vi "GSP_GUI_user.vi"(4 "error in":errorcluster, 7 "User File":path) -> (0 "error out":errorcluster, 1 "User Type":T1, 2 "Canceled?":bool)   [LabVIEW 2015]
doc: "A login GUI that reads and validates from the supplied user INI file"
uses:
  GUI_states.ctl
  GSP_GUI_global.vi
panel:
  out "Status":string
  in  "OK Button":bool
  in  "Password":string
  in  "Known Users":u16(ring) items=["barlow", "operators", "fraga", "rosteen", "clemens", "heathcote", "points", "unc", "msu", "brazil", "noao"]
  # "Welcome to the Goodman Spectrograph Control System. Please Select your username to the right or enter a a new name and press \"OK\""
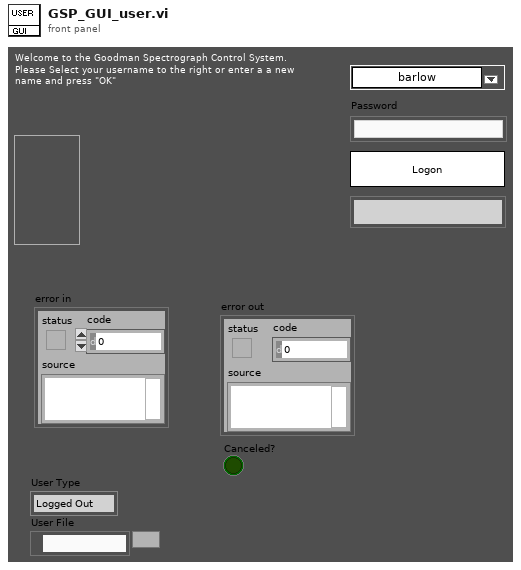
[diagram p1: front panel]
types:
  T1 = typedef "GUI_states.ctl" = enum16{"Logged Out", "Observer", "Operator", "Engineer"}
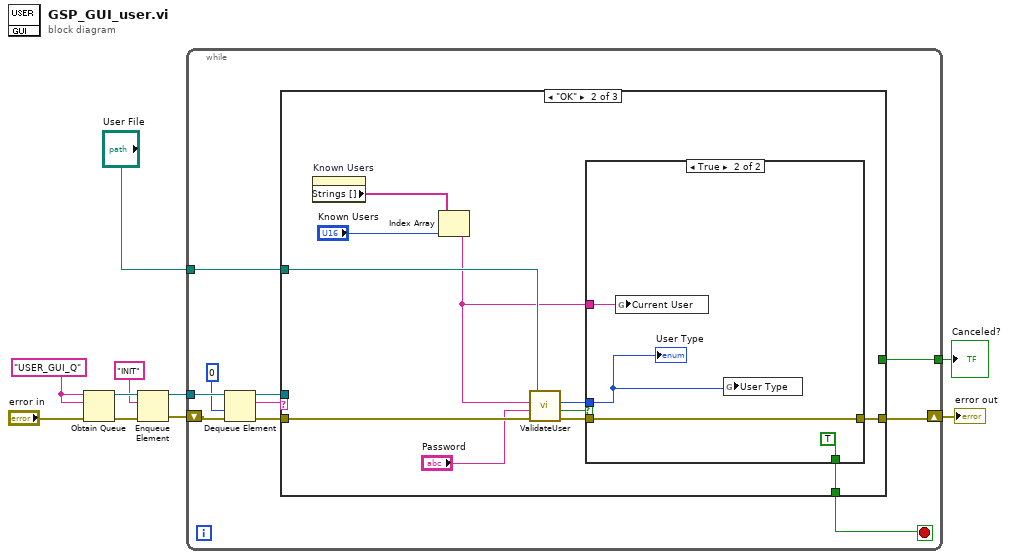
[diagram p0: block diagram]
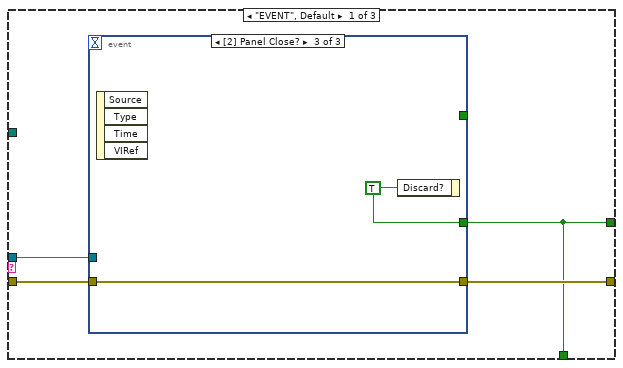
[diagram p2: hidden frame]
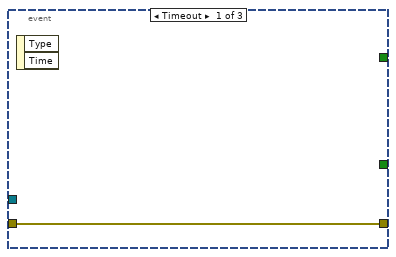
[diagram p3: hidden frame]
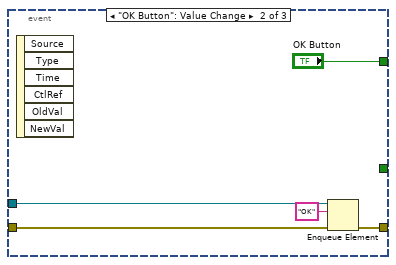
[diagram p4: hidden frame]
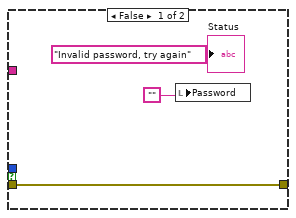
[diagram p5: hidden frame]
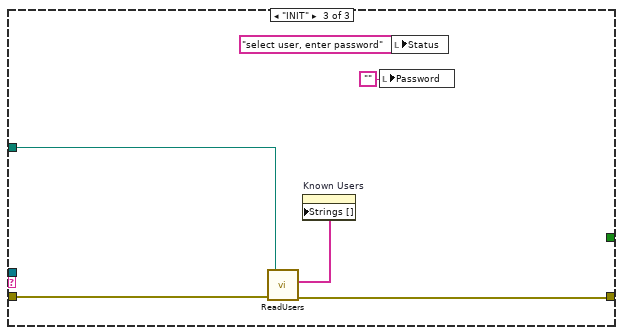
[diagram p6: hidden frame]
diagram:
  w6 = "USER_GUI_Q" ("name (unnamed)")
  n1 = Obtain Queue(name (unnamed)=w6, element data type=w6, error in (no error)="error in") -> (queue out=w10:refnum<queue>, error out=w9:errorcluster)  [unwired: 2 in, 1 out]
  n2 = Enqueue Element(queue=w10, element="INIT", error in (no error)=w9) -> (queue out=w8:refnum<queue>, error out=w4:errorcluster)  [unwired: 1 in, 1 out]
  n3 = while {
    tunnel: w8 -> [w20]
    shift-right: [w14] -> w3
    shift-left: w4 -> [w15]
    tunnel: [w12] -> w2
    tunnel: "User File" -> [w11]
    stop <- w13 stop-if-true
    n4 = Dequeue Element(queue=w20, timeout in ms (-1)=0, error in (no error)=w15) -> (queue out=w18:refnum<queue>, element=w19:string, error out=w17:errorcluster)  [unwired: 1 out]
    n5 = case shown="\"OK\"" w19 {
      tunnel: w18 -> [w23 _ _]
      tunnel: w17 -> [w24 w42 w56]
      tunnel: [w22 w34 w55] -> w14
      tunnel: [w21 w33 _] -> w13
      tunnel: [w21 _ _] -> w12
      tunnel: w11 -> [_ w40 w51]
      frame "EVENT", Default {
        n6 = event shown="[2] Panel Close?" {
          selector: _ -> [_ _ _]
          dyn-events: _ -> [_ _ _]
          timeout: _ -> [_ _ _]
          tunnel: w24 -> [w25 w27 w32]
          tunnel: w23 -> [_ w28 _]
          tunnel: [w25 w29 w32] -> w22
          tunnel: [_ "OK Button" _] -> _
          tunnel: [_ _ w31] -> w21
          event Timeout {
            n7 = event-data() -> ()  [unwired: 1 in, 2 out]
          }
          event "OK Button": Value Change {
            n8 = event-data() -> ()  [unwired: 1 in, 6 out]
            n9 = Enqueue Element(queue=w28, element="OK", error in (no error)=w27) -> (error out=w29:errorcluster)  [unwired: 1 in, 2 out]
          }
          event Panel Close? {
            w31 = TRUE
            n10 = event-data() -> ()  [unwired: 1 in, 4 out]
            n11 = event-data("Discard?"=w31) -> ()  [unwired: 1 in, 1 out]
          }
        }
      }
      frame "OK" {
        n12 = property on="Known Users" class="Ring (strict)"() -> ("Strings []"=w43:string[])  [unwired: 2 in, 2 out]
        n13 = Index Array(array=w43, index="Known Users") -> (element=w36:string)
        n14 = call "ValidateUser.vi"("error in (no error)"=w42, "password"="Password", "username"=w36, "configuration file path"=w40) -> ("error out"=w37:errorcluster, "Valid Password?"=w38:bool, "User Type"=w35:T1)  [unwired: 1 out]
        n15 = case shown="True" w38 {
          tunnel: w37 -> [w45 w49]
          tunnel: w36 -> [_ w50]
          tunnel: w35 -> [_ w47]
          tunnel: [w45 w49] -> w34
          tunnel: [_ TRUE] -> w33
          frame False {
            n16 = local write "Password"("") -> ()
            "Status" <- "Invalid password, try again" ("Status")
          }
          frame True {
            n17 = global write "GSP_GUI_global.vi" "Current User"(w50) -> ()
            n18 = global write "GSP_GUI_global.vi" "User Type"(w47) -> ()
            "User Type" <- w47
          }
        }
      }
      frame "INIT" {
        n19 = call "ReadUsers.vi"("error in (no error)"=w56, "configuration file path"=w51) -> ("error out"=w55:errorcluster, "known users"=w54:string[])  [unwired: 3 in, 1 out]
        n20 = property on="Known Users" class="Ring (strict)"("Strings []"=w54) -> ()  [unwired: 2 in, 2 out]
        n21 = local write "Password"("") -> ()
        n22 = local write "Status"("select user, enter password" ("Status")) -> ()
      }
    }
  }
  "error out" <- w3
  "Canceled?" <- w2
